vi "nominal run create.vi"(0 "client":i32, 1 "end_ms":dbl, 2 "out_run":i32, 5 "name":string, 7 "description":string, 9 "start_ms":dbl, 11 "error in (no error)":errorcluster, 12 "has_end":bool) -> (4 "out_run out":i32, 6 "function return":i32, 15 "error out":errorcluster)   [LabVIEW 2020, in "client.lvlib"]
doc: "int32_t nominal_run_create(int32_t client,\n const char *name,\n const char *description,\n double start_ms,\n double end_ms,\n bool has_end,\n int32_t *out_run);"
uses:
  client.lvlib
  bin/nominalClient_64.dll
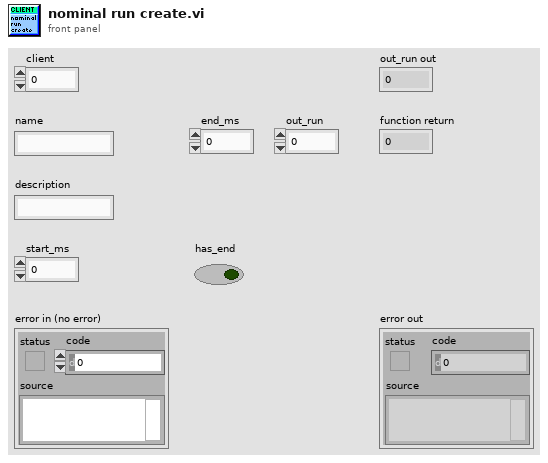
[diagram p1: front panel]
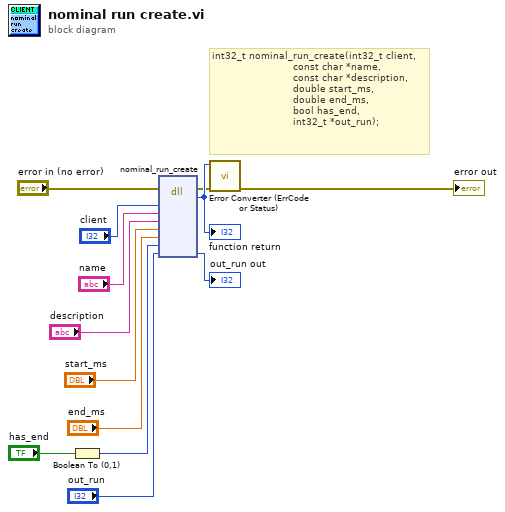
[diagram p0: block diagram]
diagram:
  # "int32_t nominal_run_create(int32_t client,\n                           const char *name,\n                           const char *description,\n                           double start_ms,\n                           double end_ms,\n                           bool has_end,\n                           int32_t *out_run);"
  n1 = Boolean To (0,1)(Boolean="has_end") -> (0, 1=w6:i16)
  n2 = dll-call lib="C:/code/labview-client-rs/lv_src/bin/nominalClient_*.*" fn="nominal_run_create"(error in="error in (no error)", "client"="client", "name"="name", "description"="description", "start_ms"="start_ms", "end_ms"="end_ms", "has_end"=w6, "out_run"="out_run") -> (error out=w2:errorcluster, w13:i32, "out_run"=→"out_run out":i32)  [unwired: 8 in, 1 out]
  "function return" <- w13
  n3 = call "Error Converter (ErrCode or Status).vi"("error in (no error)"=w2, "error code"=w13) -> ("error out"=→"error out":errorcluster)  [unwired: 9 in]
